vi "MW power meter over time.vi"() -> ()   [LabVIEW 2012]
uses:
  <vilib>/Utility/file.llb/Write To Spreadsheet File (DBL).vi
panel:
  in  "file path (dialog if empty)":path
  out "Elapsed Time (s)":dbl
  out "Waveform Graph":ext[](graph)
  in  "stop":bool
  out "frequency (Hz)":ext format="%.1f"
  out "Power dbm":ext format="%.1f"
  in  "GPIB Address":string="19"
  in  "band (1-26.5 GHz:20)":i32(ring)=2
  in  "resolution (1 Hz:1)":i32(ring)=1 items=["0.1 Hz", "1 Hz", "10 Hz", "100 Hz", "1 KHz", "10 KHz", "100 KHz", "1 MHz", "10 MHz", "100 MHz", "1 GHz"]
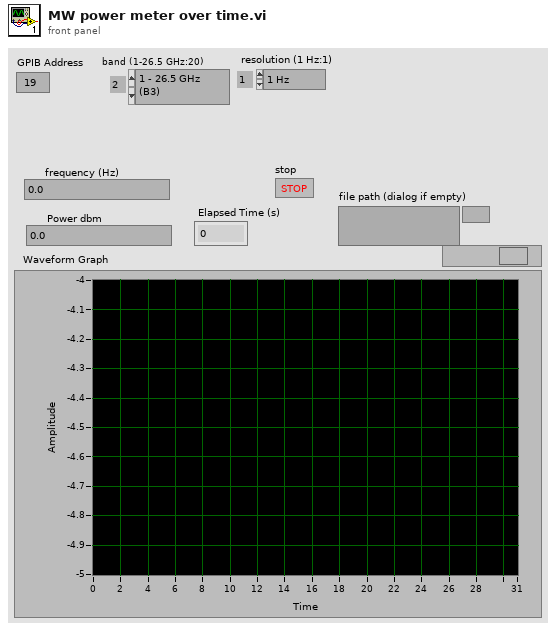
[diagram p1: front panel]
types:
  T1 = cluster{"source lock":bool, "lock frequency (Hz)":ext, "coarse tune":bool}
  T2 = cluster{"power\nmeter":bool, bool, "Power Offset":ext}
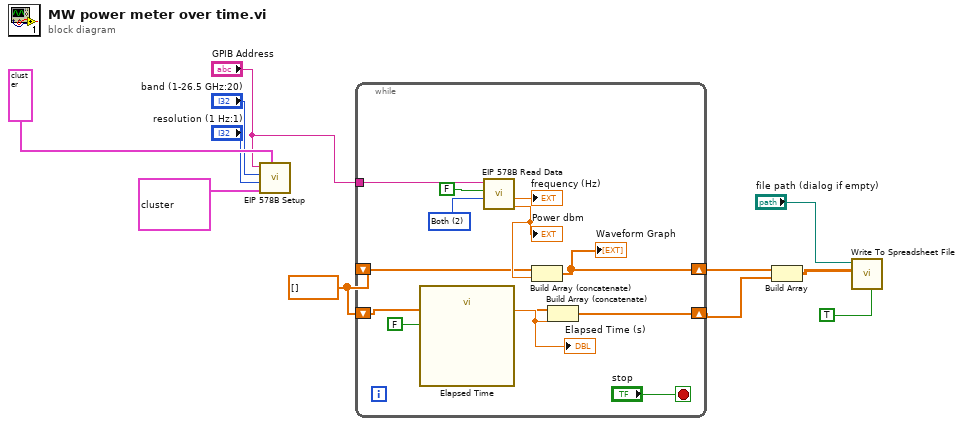
[diagram p0: block diagram]
diagram:
  w6 = ext[] []
  n1 = call "EIP 578B Setup.vi"("GPIB Address"="GPIB Address", "band (1-26.5 GHz:20)"="band (1-26.5 GHz:20)", "resolution (1 Hz:1)"="resolution (1 Hz:1)", "source locking"=T1 {"source lock"=FALSE, "lock frequency (Hz)"=1000000000.0, "coarse tune"=FALSE}, "power meter"=T2 {"power\nmeter"=TRUE, TRUE, "Power Offset"=0.0}) -> ()  [unwired: 1 in, 2 out]
  n2 = while {
    tunnel: "GPIB Address" -> [w20]
    shift-right: [w18] -> w5
    shift-left: w6 -> [w16]
    shift-right: [w15] -> w4
    shift-left: w6 -> [w13]
    stop <- "stop" stop-if-true
    w23 = 2 items=["Frequency", "Power", "Both"] ("output mode (freq:0)")
    n3 = call "Elapsed Time"("Auto Reset"=FALSE) -> ("Elapsed Time (s)"=w14:dbl)  [unwired: 11 in, 7 out]
    "Elapsed Time (s)" <- w14
    n4 = call "EIP 578B Read Data.vi"("output mode (freq:0)"=w23, "fast (T=active)"=FALSE, "GPIB"=w20) -> ("Power (dBm)"=w17:ext, "frequency (Hz)"=→"frequency (Hz)":ext)  [unwired: 1 in, 2 out]
    "Power dbm" <- w17
    n5 = Build Array (concatenate)(w16, w17) -> (w18:ext[])
    "Waveform Graph" <- w18
    n6 = Build Array (concatenate)(w13, w14) -> (w15:ext[])
  }
  n7 = Build Array(w5, w4) -> (w3:ext[][])
  n8 = call-poly <vilib>:"Write To Spreadsheet File.vi"("transpose? (no:F)"=TRUE, "2D data"=w3, "file path (dialog if empty)"="file path (dialog if empty)") -> ()  [unwired: 5 in, 1 out]
